vi "EndIf.vi"(8 "False In":T1={"Port"="", "All Code"="Hi"}, 11 "True In":T1) -> (3 "Data Out":T1={"Port"="", "All Code"="Hi"})   [LabVIEW 2016]
uses:
  uPythonX/PythonData.ctl
  uPythonX/uPythonX.xctl
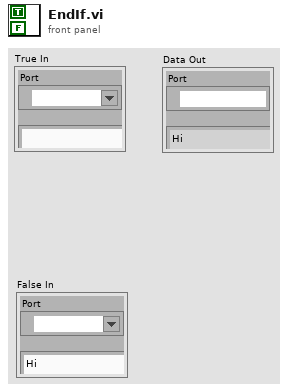
[diagram p1: front panel]
types:
  T1 = typedef "uPythonX.xctl/PythonData.ctl" = cluster{"Port":refnum<visa-resource-name>, "All Code":string}
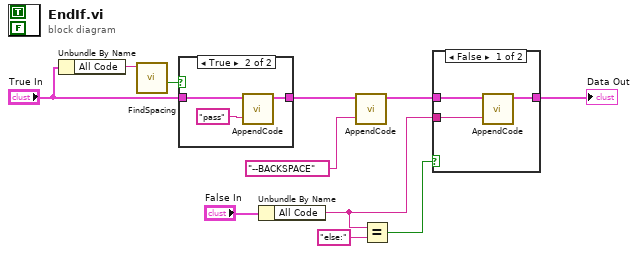
[diagram p0: block diagram]
diagram:
  n1 = Unbundle By Name("True In") -> ("All Code"=w7:string)
  n2 = call "FindSpacing.vi"("All Code"=w7) -> ("indent?"=w4:bool)  [unwired: 8 in, 2 out]
  n3 = case shown="True" w4 {
    tunnel: "True In" -> [w12 w15]
    tunnel: [w12 w14] -> w5
    frame False {
    }
    frame True {
      n4 = call "AppendCode.vi"("New Code"="pass", "Data In"=w15) -> ("Data Out"=w14:T1)  [unwired: 9 in]
    }
  }
  n5 = Unbundle By Name("False In") -> ("All Code"=w3:string)
  n6 = call "AppendCode.vi"("New Code"="--BACKSPACE", "Data In"=w5) -> ("Data Out"=w9:T1)  [unwired: 9 in]
  n7 = Equal?(x=w3, y="else:") -> (x = y?=w1:bool)
  n8 = case shown="False" w1 {
    tunnel: w9 -> [w18 w19]
    tunnel: [w17 w19] -> w8
    tunnel: w3 -> [w16 _]
    frame False {
      n9 = call "AppendCode.vi"("New Code"=w16, "Data In"=w18) -> ("Data Out"=w17:T1)  [unwired: 9 in]
    }
    frame True {
    }
  }
  "Data Out" <- w8
